vi "(SubVI)Haptic Vibration Scope.vi"() -> ()   [LabVIEW 2020]
uses:
  Controls/(Ctrl)Scope_Peak to Peak.ctl
  Controls/(Ctrl)Scope_Sensor Axis.ctl
  Controls/(Ctrl)Scope_Queue Cluster.ctl
  Controls/(Ctrl)Scope_Command Enum.ctl
  Control Data/Controls/(Ctrl)Control Data_Save or Load Control Data_Function.ctl
  Mode Event/Controls/(Ctrl)Mode Event_FGV Function.ctl
  <vilib>/Utility/miscctls.llb/LVPointTypeDef.ctl
  Mode Event/Controls/(Ctrl)Mode Event_Event Type.ctl
  Serial/Controls/(Ctrl)Serial_FGV Function.ctl
  Controls/(Ctrl)Scope_Mode.ctl
  04adf9c7-eebe-4733-9548-b5fb3f9c431f.vi
  aeb30a4b-5dd8-45a1-ad12-ebdf0f741a30.vi
  Variables/(Var)System Variables.vi
panel:
  in  "Graph_Legend Blind S3":string
  in  "Graph_Legend Blind S2":string
  in  "Graph_Legend Blind S1":string
  in  "Scope_Stop":bool
  in  "Mode":enum32{"Auto Playback", "Scope Mode"}(tab)=enum."Scope Mode"
  in  "Auto_Record Time":dbl(ring)=0.1 caption="Record Time" items=["0.1sec"=0.1, "0.2sec"=0.2, "0.3sec"=0.3, "0.4sec"=0.4, "0.5sec"=0.5]
  in  "Auto_Start":bool
  in  "Scope_Start":bool
  in  "Scope_Trig Type":enum16{"None", "Repeat", "Single"}(ring) caption="Trigger"
  in  "Scope_Trig Ch":i32(ring)=-1 caption="Channel" items=["All Channel"=-1, "Sensor 1 - X"=0, "Sensor 1 - Y"=1, "Sensor 1 - Z"=2, "Sensor 2 - X"=3, "Sensor 2 - Y"=4, "Sensor 2 - Z"=5, "Sensor 3 - X"=6, "Sensor 3 - Y"=7, "Sensor 3 - Z"=8]
  in  "Scope_Trig Level":dbl=1.0 caption="Level" min=-16.0 max=16.0 format="%#_gg"
  in  "Scope_Trig Edge":enum16{"Rising", "Falling"}(ring) caption="Edge"
  in  "Scope_Pre-trigger":dbl(ring)=0.1 caption="Pre-trigger" items=["0%"=0.0, "10%"=0.1, "20%"=0.2, "30%"=0.3, "40%"=0.4, "50%"=0.5, "60%"=0.6, "70%"=0.7, "80%"=0.8, "90%"=0.9, "100%"=1.0]
  in  "Scope_Record Time":dbl(ring)=1.0 caption="Record Time" items=["0.1sec"=0.1, "0.2sec"=0.2, "0.3sec"=0.3, "0.4sec"=0.4, "0.5sec"=0.5, "0.6sec"=0.6, "0.7sec"=0.7, "0.8sec"=0.8, "0.9sec"=0.9, "1sec"=1.0, "2sec"=2.0, "3sec"=3.0, "4sec"=4.0, "5sec"=5.0, "6sec"=6.0, "7sec"=7.0, "8sec"=8.0, "9sec"=9.0, "10sec"=10.0]
  out "Graph":dbl[][](graph)
  out "Overrun Cnt":i32
  out "Latency":i32
  out "Graph_PP":T1 {"S3_Value" format="%#_gg"; "S2_Value" format="%#_gg"; "S1_Value" format="%#_gg"}
  in  "Graph_Auto Scale_Y":enum32{"선택 없음", "±16 g", "Auto Scale"}(radio)=enum."±16 g" caption="Y (Acc) -"
  in  "Graph_Auto Scale_X":bool=TRUE
  # "Haptic Vibration Scope"
  # "Sensor 1"
  # "Sensor 2"
  # "Sensor 3"
  # "Graph Scale"
  # "P·P"
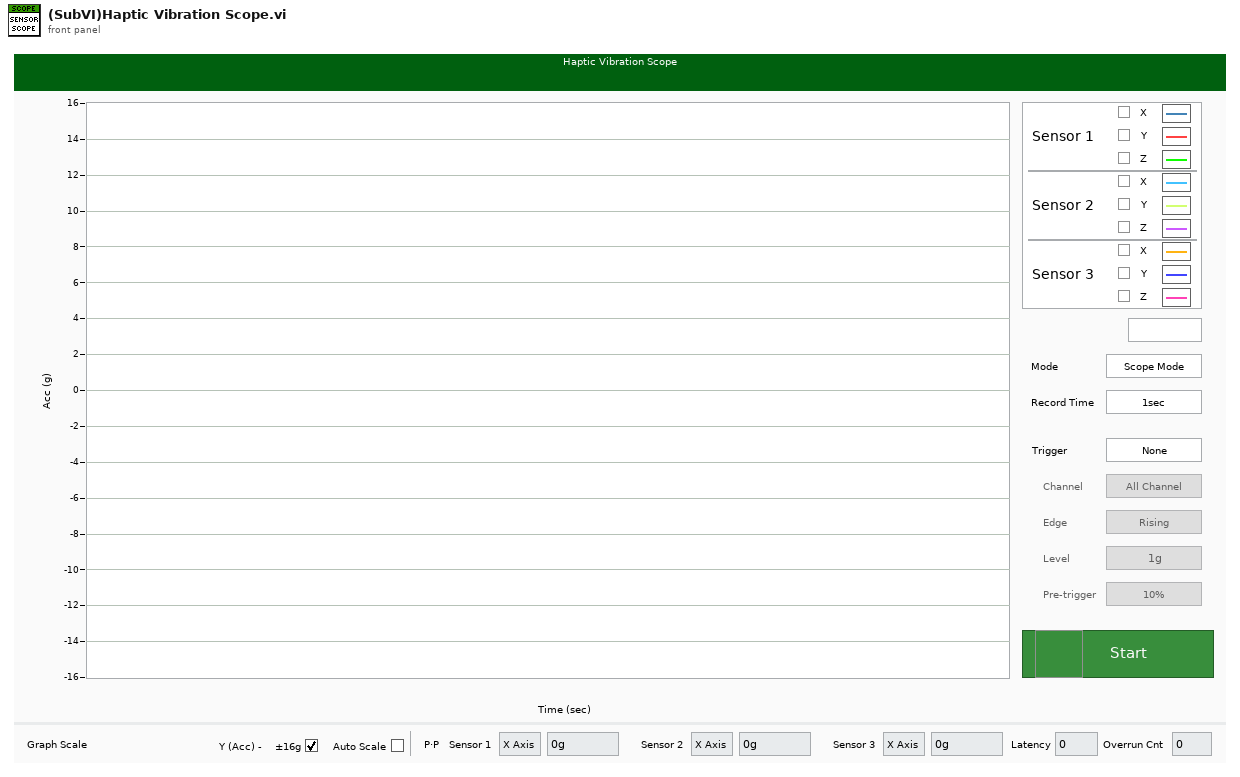
[diagram p1: front panel]
types:
  T1 = typedef "(Ctrl)Scope_Peak to Peak.ctl" = cluster{"S1_Axis":T2, "S1_Value":dbl, "S2_Axis":T2, "S2_Value":dbl, "S3_Axis":T2, "S3_Value":dbl}
  T2 = typedef "(Ctrl)Scope_Sensor Axis.ctl" = enum16{"X Axis", "Y Axis", "Z Axis"}
  T3 = enum8{"Enabled", "Disabled", "Disabled and Grayed Out"}
  T4 = typedef "(Ctrl)Mode Event_FGV Function.ctl" = enum16{"Init", "Get Event Ref", "Gen Event", "Destroy"}
  T5 = typedef "(Ctrl)Control Data_Save or Load Control Data_Function.ctl" = enum16{"Save", "Load"}
  T6 = typedef "(Ctrl)Scope_Queue Cluster.ctl" = cluster{"Command":T7, "Data":variant}
  T7 = typedef "(Ctrl)Scope_Command Enum.ctl" = enum16{"Scope_Start", "Scope_Receive", "Scope_I2C", "Scope_Stop"}
  T8 = typedef "LVPointTypeDef.ctl" = cluster{"Horizontal":i16, "Vertical":i16}
  T9 = typedef "Haptic IC.lvclass/(Ctrl)IC Type.ctl" = enum8{"DW7800", "DW7802", "DW7912", "DW7914"}
  T10 = enum32{"Page Enabled", "Page Disabled", "Page Disabled & Grayed"}
  T11 = typedef "(Ctrl)Mode Event_Event Type.ctl" = enum16{"RTP Play", "RTP Stop", "Scope Start", "Scope Stop"}
  T12 = typedef "(Ctrl)Scope_Mode.ctl" = enum8{"Auto Trigger Mode", "Continuous Mode"}
  T13 = typedef "(Ctrl)Serial_FGV Function.ctl" = enum16{"Initialize", "Read", "Read All", "Write", "Flush Buffer", "Get Ref.", "Close"}
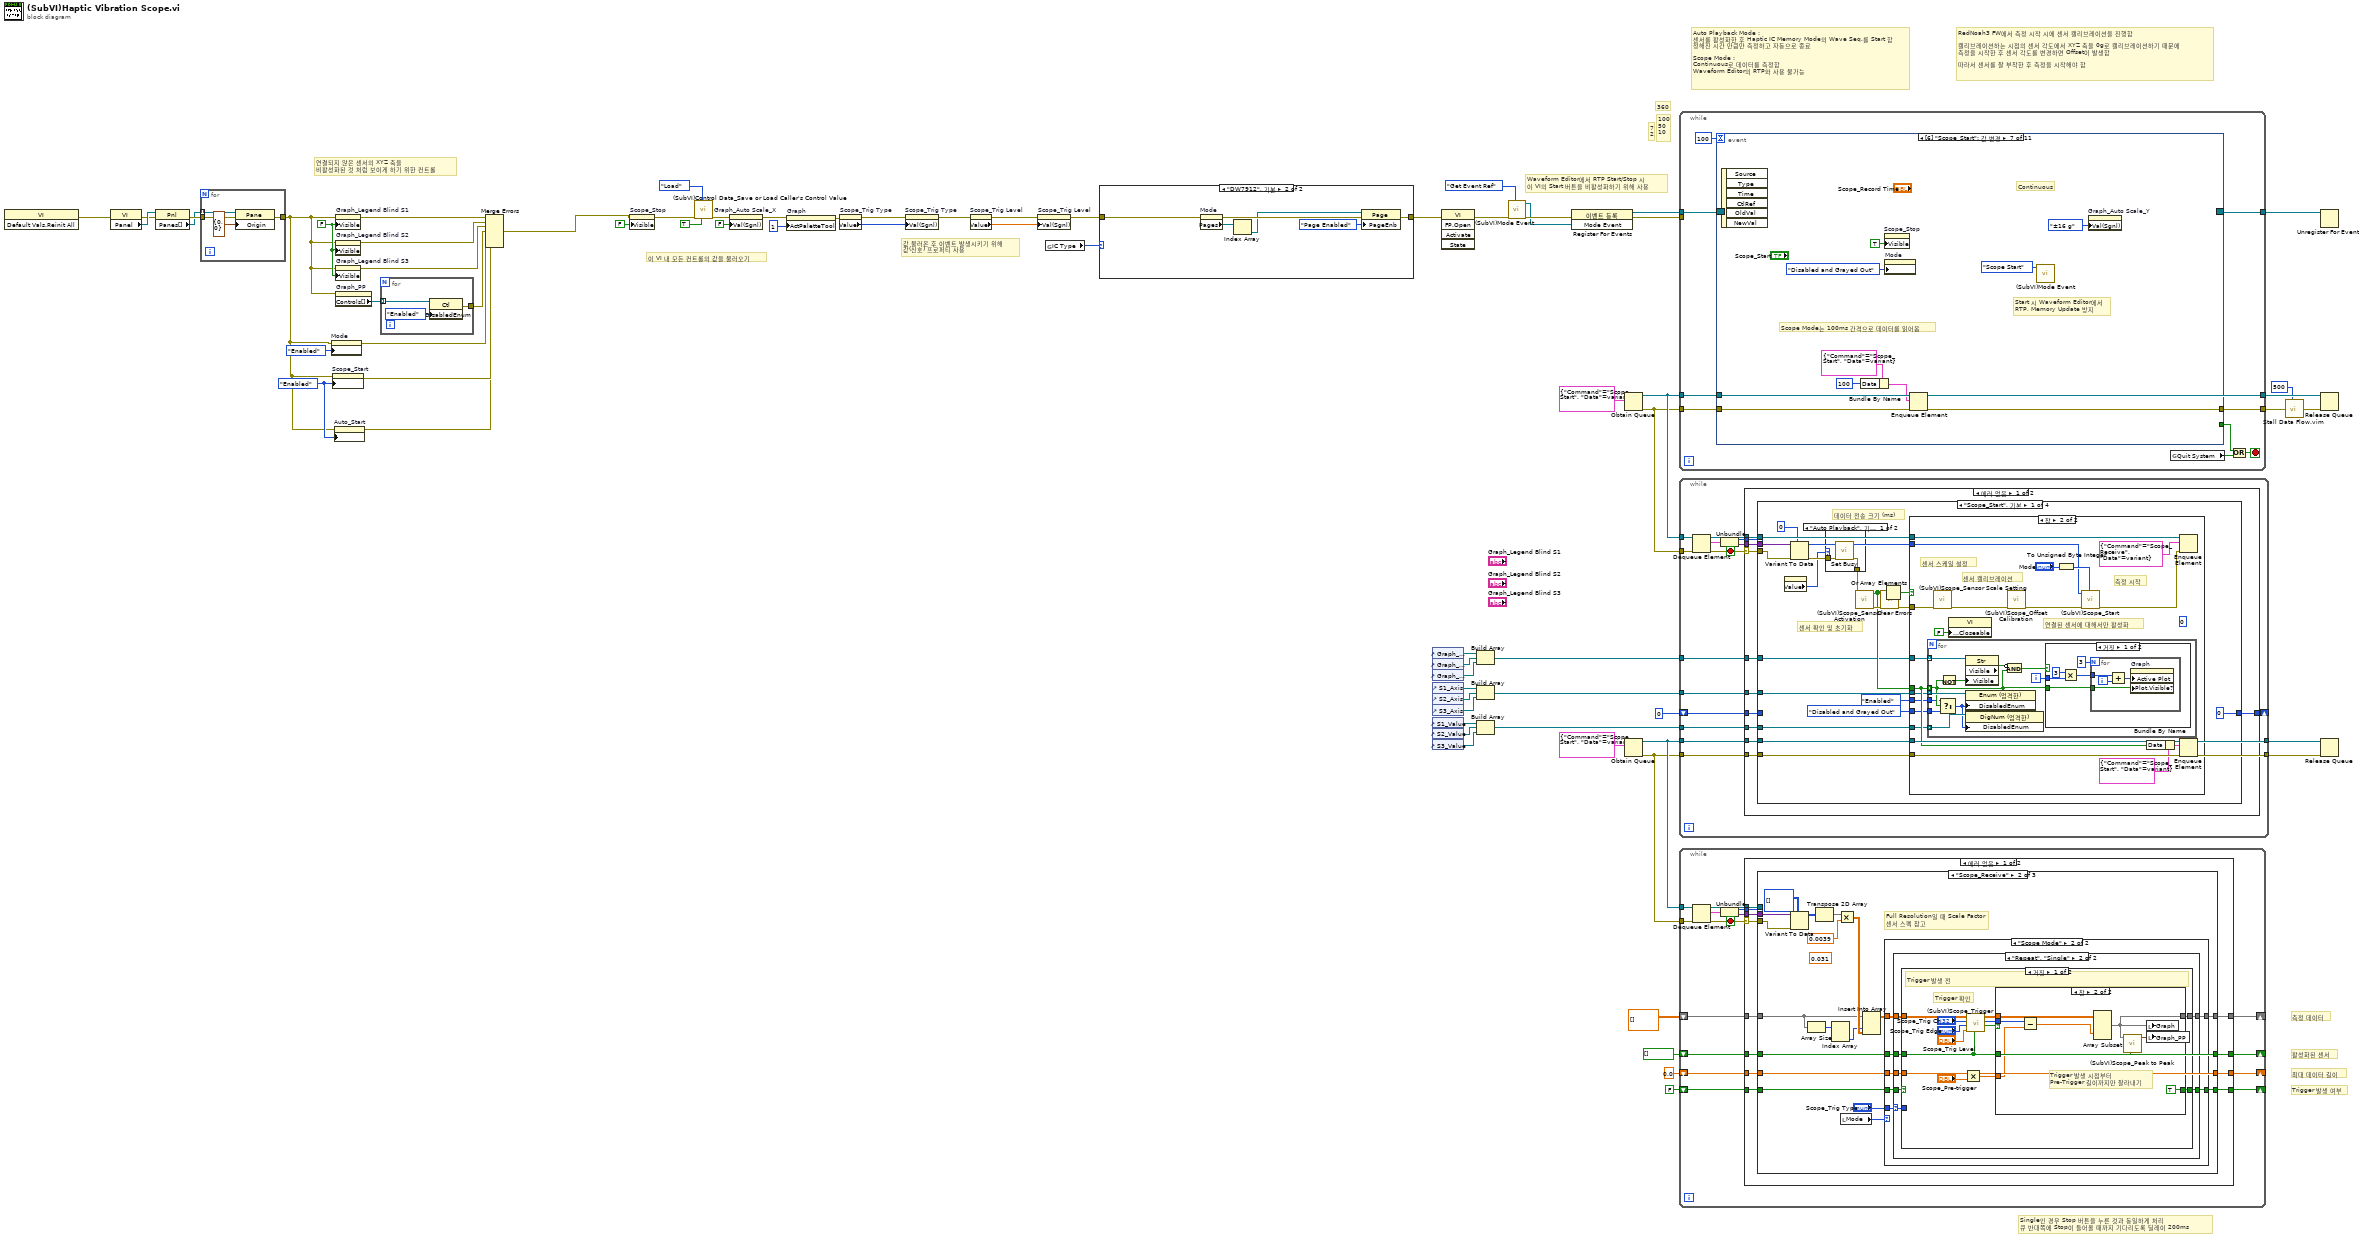
[diagram p0: block diagram]
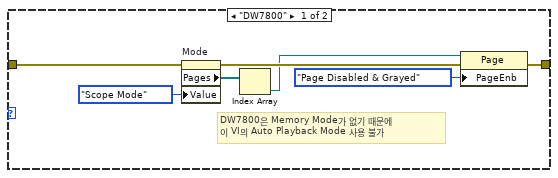
[diagram p2: hidden frame]
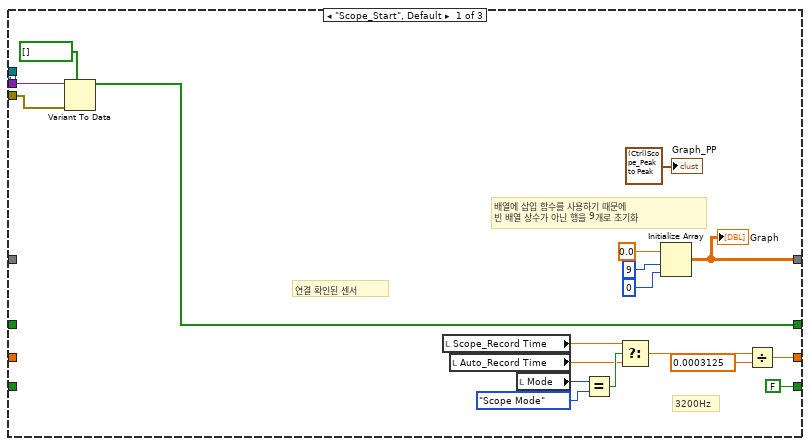
[diagram p3: hidden frame]
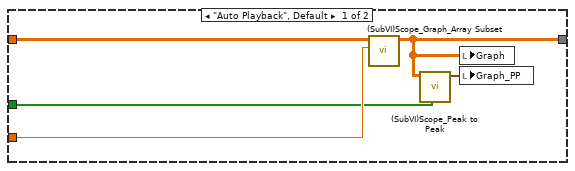
[diagram p4: hidden frame]
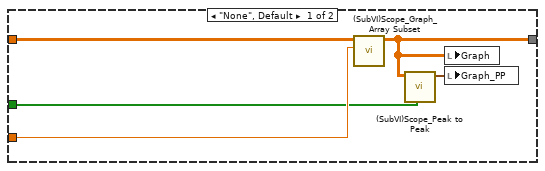
[diagram p5: hidden frame]
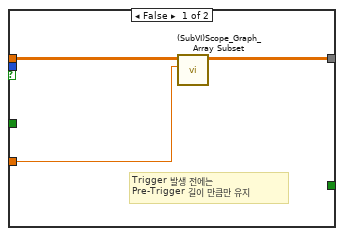
[diagram p6: hidden frame]
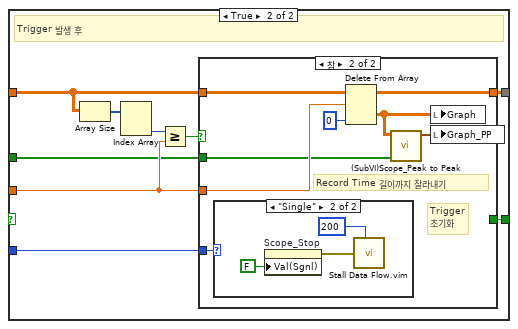
[diagram p7: hidden frame]
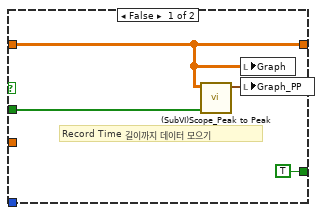
[diagram p8: hidden frame]
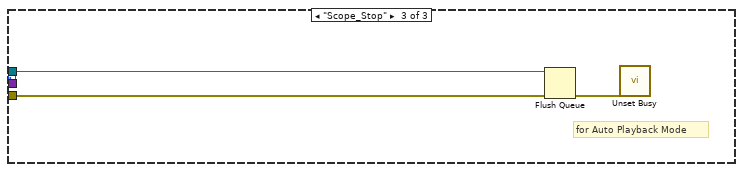
[diagram p10: hidden frame]
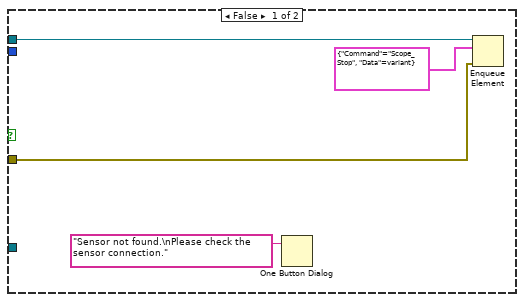
[diagram p13: hidden frame]
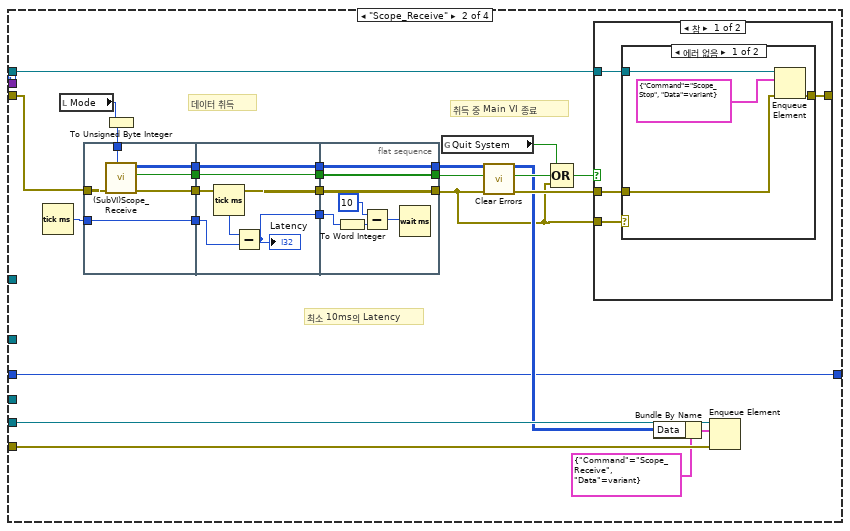
[diagram p15: hidden frame]
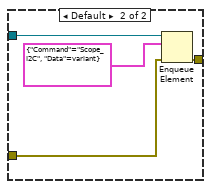
[diagram p16: hidden frame]
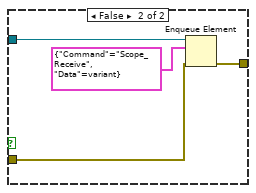
[diagram p17: hidden frame]
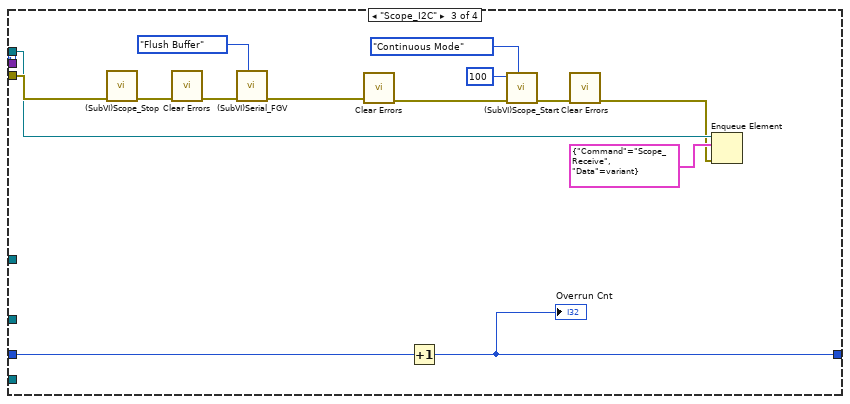
[diagram p18: hidden frame]
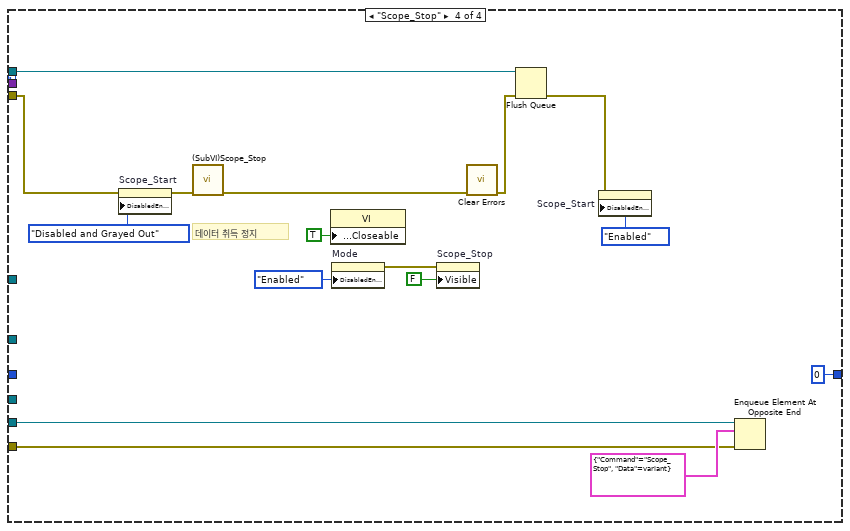
[diagram p19: hidden frame]
diagram:
  w10 = T3."Enabled" ("비활성화")
  w31 = FALSE ("보이기")
  # "7\n2"
  # "360"
  # "100\n50\n10"
  # "Single인 경우 Stop 버튼을 누른 것과 동일하게 처리\n큐 반대쪽에 Stop이 들어올 때까지 기다리도록 딜레이 200ms"
  # "Trigger 발생 여부"
  # "최대 데이터 길이"
  # "활성화된 센서"
  # "측정 데이터"
  # "RedNoah3 FW에서 측정 시작 시에 센서 캘리브레이션을 진행함\n\n캘리브레이션하는 시점의 센서 각도에서 XYZ 축을 0g로 캘리브레이션하기 때문에\n측정을 시작한 후 센서 각도를 변경하면 Offset이 발생함\n\n따라서 센서를 잘 부착한 후 측정을 시작해야 함"
  # "Auto Playback Mode : \n센서를 활성화한 후 Haptic IC Memory Mode의 Wave Seq.를 Start 함\n정해진 시간 만큼만 측정하고 자동으로 종료\n\nScope Mode : \nContinuous로 데이터를 측정함\nWaveform Editor의 RTP와 사용 불가능"
  # "Waveform Editor에서 RTP Start/Stop 시\n이 VI의 Start 버튼을 비활성화하기 위해 사용"
  # "값 불러온 후 이벤트 발생시키기 위해\n값(신호) 프로퍼티 사용"
  # "이 VI 내 모든 컨트롤의 값을 불러오기"
  # "연결되지 않은 센서의 XYZ 축을 \n비활성화된 것 처럼 보이게 하기 위한 컨트롤"
  n1 = invoke class="VI" method="Default Vals.Reinit All"() -> (error out=w35:errorcluster)  [unwired: 3 in, 2 out]
  n2 = property class="VI"(error in=w35) -> (error out=w34:errorcluster, "Panel"=w36:refnum<vi>)  [unwired: 1 in, 1 out]
  n3 = property class="Pnl"(reference=w36, error in=w34) -> (error out=w33:errorcluster, "Panes[]"=w32:refnum<vi>[])  [unwired: 1 out]
  n4 = for {
    tunnel: w33 -> [w75]
    tunnel: w32 -> [w74] mode=indexing
    tunnel: [w72] -> w9
    n5 = property class="Pane"(reference=w74, error in=w75, "Origin"=T8 {"Horizontal"=0, "Vertical"=0} ("원점")) -> (error out=w72:errorcluster)  [unwired: 1 out]
  }
  n6 = property on="Mode" class="TabCtl (엄격한)"(error in=w9, "DisabledEnum"=T3."Enabled" ("비활성화")) -> (error out=w8:errorcluster)  [unwired: 1 in, 1 out]
  n7 = property on="Scope_Start" class="Bool"(error in=w9, "DisabledEnum"=w10) -> (error out=w7:errorcluster)  [unwired: 1 in, 1 out]
  n8 = property on="Auto_Start" class="Bool"(error in=w9, "DisabledEnum"=w10) -> (error out=w6:errorcluster)  [unwired: 1 in, 1 out]
  n9 = property on="Graph_Legend Blind S1" class="Str"(error in=w9, "Visible"=w31) -> (error out=w30:errorcluster)  [unwired: 1 in, 1 out]
  n10 = property on="Graph_Legend Blind S2" class="Str"(error in=w9, "Visible"=w31) -> (error out=w29:errorcluster)  [unwired: 1 in, 1 out]
  n11 = property on="Graph_Legend Blind S3" class="Str"(error in=w9, "Visible"=w31) -> (error out=w28:errorcluster)  [unwired: 1 in, 1 out]
  n12 = property on="Graph_PP" class="Clust (엄격한)"(error in=w9) -> ("Controls[]"=w15:refnum<vi>[])  [unwired: 1 in, 2 out]
  n13 = for {
    tunnel: w15 -> [w78] mode=indexing
    tunnel: [w76] -> w14
    n14 = property class="Ctl"(reference=w78, "DisabledEnum"=T3."Enabled" ("비활성화")) -> (error out=w76:errorcluster)  [unwired: 1 in, 1 out]
  }
  n15 = Merge Errors(w30, w29, w28, w14, w8, w6, w7) -> (w1:errorcluster)
  n16 = property on="Scope_Stop" class="Bool (엄격한)"(error in=w1, "Visible"=FALSE ("보이기")) -> (error out=w64:errorcluster)  [unwired: 1 in, 1 out]
  n17 = call "(SubVI)Control Data_Save or Load Caller's Control Value.vi"("Common?"=TRUE, "Function"=(Ctrl)Control_Data_Save_or_Load_Control_Data_Function."Load", "error in (no error)"=w64) -> ("error out"=w13:errorcluster)  [unwired: 8 in]
  n18 = property on="Graph_Auto Scale_X" class="Bool (엄격한)"(error in=w13, "Val(Sgnl)"=FALSE ("값(신호)")) -> (error out=w5:errorcluster)  [unwired: 1 in, 1 out]
  n19 = property on="Graph" class="WFGraph (엄격한)"(error in=w5, "ActPaletteTool"=1 ("팔레트:활성 도구")) -> (error out=w4:errorcluster)  [unwired: 1 in, 1 out]
  n20 = property on="Scope_Trig Type" class="Enum (엄격한)"(error in=w4) -> (error out=w50:errorcluster, "Value"=w49:enum16{"None", "Repeat", "Single"})  [unwired: 1 in, 1 out]
  n21 = property on="Scope_Trig Type" class="Enum (엄격한)"(error in=w50, "Val(Sgnl)"=w49) -> (error out=w48:errorcluster)  [unwired: 1 in, 1 out]
  n22 = property on="Scope_Trig Level" class="DigNum (엄격한)"(error in=w48) -> (error out=w46:errorcluster, "Value"=w47:dbl)  [unwired: 1 in, 1 out]
  n23 = property on="Scope_Trig Level" class="DigNum (엄격한)"(error in=w46, "Val(Sgnl)"=w47) -> (error out=w45:errorcluster)  [unwired: 1 in, 1 out]
  n24 = global read "(Var)System Variables.vi" "IC Type"() -> (w51:T9)
  n25 = case shown="\"DW7912\", 기본" w51 {
    tunnel: [w82 w88] -> w63
    tunnel: w45 -> [w81 w87]
    frame "DW7800" {
      # "DW7800은 Memory Mode가 없기 때문에\n이 VI의 Auto Playback Mode 사용 불가"
      n26 = property on="Mode" class="TabCtl (엄격한)"(error in=w81, "Value"=enum32{"Auto Playback", "Scope Mode"}."Scope Mode" ("Mode")) -> (error out=w84:errorcluster, "Pages"=w85:refnum<vi>[])  [unwired: 1 in, 1 out]
      n27 = Index Array(array=w85) -> (element=w83:refnum<vi>)  [unwired: 1 in]
      n28 = property class="Page"(reference=w83, error in=w84, "PageEnb"=T10."Page Disabled & Grayed" ("페이지 활성화 상태")) -> (error out=w82:errorcluster)  [unwired: 1 out]
    }
    frame "DW7912", Default {
      n29 = property on="Mode" class="TabCtl (엄격한)"(error in=w87) -> (error out=w90:errorcluster, "Pages"=w91:refnum<vi>[])  [unwired: 1 in, 1 out]
      n30 = Index Array(array=w91) -> (element=w89:refnum<vi>)  [unwired: 1 in]
      n31 = property class="Page"(reference=w89, error in=w90, "PageEnb"=T10."Page Enabled" ("페이지 활성화 상태")) -> (error out=w88:errorcluster)  [unwired: 1 out]
    }
  }
  n32 = control-ref of="Graph_Legend Blind S1"() -> (w27:refnum<vi>)
  n33 = control-ref of="Graph_Legend Blind S2"() -> (w26:refnum<vi>)
  n34 = control-ref of="Graph_Legend Blind S3"() -> (w25:refnum<vi>)
  n35 = control-ref of="S1_Axis"() -> (w23:refnum<vi>)
  n36 = control-ref of="S2_Axis"() -> (w22:refnum<vi>)
  n37 = control-ref of="S3_Axis"() -> (w21:refnum<vi>)
  n38 = control-ref of="S1_Value"() -> (w20:refnum<vi>)
  n39 = control-ref of="S2_Value"() -> (w19:refnum<vi>)
  n40 = control-ref of="S3_Value"() -> (w18:refnum<vi>)
  n41 = invoke class="VI" method="FP.Open"(error in=w63) -> (error out=w71:errorcluster)  [unwired: 4 in, 4 out]
  n42 = Build Array(w27, w26, w25) -> (w24:refnum<vi>[])
  n43 = Build Array(w23, w22, w21) -> (w17:refnum<vi>[])
  n44 = Build Array(w20, w19, w18) -> (w16:refnum<vi>[])
  n45 = call "(SubVI)Mode Event.vi"("Function (Gen)"=(Ctrl)Mode_Event_FGV_Function."Get Event Ref" ("Function"), "error in (no error)"=w71) -> ("error out"=w44:errorcluster, "Mode Event"=w40:refnum<user-event>)  [unwired: 8 in]
  n46 = register-events(error in=w44, w40) -> (reference out=w41:refnum<event-registration>, error out=w42:errorcluster)  [unwired: 1 in]
  n47 = Obtain Queue(element data type=T6 {"Command"=enum."Scope_Start", "Data"=variant} ("클러스터")) -> (queue out=w70:refnum<queue>, error out=w69:errorcluster)  [unwired: 4 in, 1 out]
  n48 = Obtain Queue(element data type=T6 {"Command"=enum."Scope_Start", "Data"=variant} ("클러스터")) -> (queue out=w58:refnum<queue>, error out=w57:errorcluster)  [unwired: 4 in, 1 out]
  n49 = while {
    tunnel: w42 -> [_]
    tunnel: w70 -> [w95]
    tunnel: w69 -> [w94]
    tunnel: [w95] -> w68
    tunnel: [w94] -> w67
    tunnel: w41 -> [w93]
    tunnel: [w92] -> w39
    stop <- w96 stop-if-true
    n50 = event shown="[6] \"Scope_Start\": 값 변경" {
      selector: w93 -> [_ _ _ _ _ _ _ _ _ _ _]
      dyn-events: [_ _ _ _ _ _ _ _ _ _ _] -> w92
      timeout: 100 -> [_ _ _ _ _ _ _ _ _ _ _]
      tunnel: [_ TRUE _ _ _ _ _ _ _ _ _] -> w97
      tunnel: w95 -> [_ _ _ _ _ w139 w148 w153 _ _ _]
      tunnel: w94 -> [w100 _ _ _ _ w132 w145 w152 _ _ _]
      tunnel: [w100 _ _ _ _ _ _ _ _ _ _] -> _
      event Timeout {
        n51 = event-data() -> ()  [unwired: 1 in, 3 out]
      }
      event Panel Close {
        # "이 VI의 모든 컨트롤의 값을 저장"
        n52 = event-data() -> ()  [unwired: 1 in, 4 out]
        n53 = call "(SubVI)Control Data_Save or Load Caller's Control Value.vi"("Common?"=TRUE, "Function"=(Ctrl)Control_Data_Save_or_Load_Control_Data_Function."Save") -> ()  [unwired: 9 in, 1 out]
      }
      event "Scope_Trig Type", "Mode": Value Change {
        # "그래프에 Trigger 타이밍, 기준 값을 커서로 표시"
        n54 = event-data() -> ()  [unwired: 1 in, 6 out]
        n55 = local read "Scope_Record Time"() -> (w107:dbl)
        n56 = local read "Auto_Record Time"() -> (w106:dbl)
        n57 = local read "Scope_Trig Type"() -> (w112:enum16{"None", "Repeat", "Single"})
        n58 = local read "Mode"() -> (w110:enum32{"Auto Playback", "Scope Mode"})
        n59 = Not Equal?(x=w112, y=enum16{"None", "Repeat", "Single"}."None") -> (x != y?=w113:bool)
        n60 = Equal?(x=w110, y=enum32{"Auto Playback", "Scope Mode"}."Scope Mode") -> (x = y?=w108:bool)
        n61 = And(x=w113, y=w108) -> (x .and. y?=w111:bool)
        n62 = Select(t=w107, s=w108, f=w106) -> (s? t:f=w105:dbl)
        n63 = property on="Graph" class="WFGraph (엄격한)"("Cursor.Visible"=w111, "XScale.Maximum"=w105, "XScale.Minimum"=0.0 ("X 스케일.범위:최소값")) -> ()  [unwired: 2 in, 2 out]
        n64 = Select(t=T3."Enabled", s=w111, f=T3."Disabled and Grayed Out") -> (s? t:f=w114:T3)
        n65 = property on="Scope_Trig Ch" class="Ring (엄격한)"("DisabledEnum"=w114) -> ()  [unwired: 2 in, 2 out]
        n66 = property on="Scope_Trig Edge" class="Enum (엄격한)"("DisabledEnum"=w114) -> ()  [unwired: 2 in, 2 out]
        n67 = property on="Scope_Trig Level" class="DigNum (엄격한)"("DisabledEnum"=w114) -> ()  [unwired: 2 in, 2 out]
        n68 = property on="Scope_Pre-trigger" class="Ring (엄격한)"("DisabledEnum"=w114) -> ()  [unwired: 2 in, 2 out]
      }
      event "Auto_Record Time", "Scope_Record Time": Value Change {
        n69 = event-data() -> ("NewVal"=w126:dbl)  [unwired: 1 in, 5 out]
        n70 = local read "Scope_Trig Type"() -> (w122:enum16{"None", "Repeat", "Single"})
        n71 = property on="Graph" class="WFGraph (엄격한)"("XScale.Maximum"=w126, "XScale.Minimum"=0.0 ("X 스케일.범위:최소값")) -> ()  [unwired: 2 in, 2 out]
        n72 = local read "Mode"() -> (w124:enum32{"Auto Playback", "Scope Mode"})
        n73 = Equal?(x=w124, y=enum32{"Auto Playback", "Scope Mode"}."Scope Mode") -> (x = y?=w120:bool)
        n74 = Not Equal?(x=w122, y=enum16{"None", "Repeat", "Single"}."None") -> (x != y?=w119:bool)
        n75 = And(x=w120, y=w119) -> (x .and. y?=w118:bool)
        n76 = case shown="참" w118 {
          frame False {
          }
          frame True {
            # "Trigger가 활성화된 경우\nRecord Time을 변경하면\n커서 위치도 변경되어야 해서\n이벤트 발생시킴"
            n77 = local read "Scope_Pre-trigger"() -> (w127:dbl)
            n78 = property on="Scope_Pre-trigger" class="Ring (엄격한)"("Val(Sgnl)"=w127) -> ()  [unwired: 2 in, 2 out]
          }
        }
      }
      event "Scope_Trig Level", "Scope_Pre-trigger": Value Change {
        # "그래프에 Trigger 타이밍, 기준 값을 커서로 표시"
        n79 = event-data() -> ()  [unwired: 1 in, 6 out]
        n80 = local read "Scope_Record Time"() -> (w130:dbl)
        n81 = local read "Scope_Pre-trigger"() -> (w129:dbl)
        n82 = local read "Scope_Trig Level"() -> (w131:dbl)
        n83 = Compound Arithmetic op=MULTIPLY(w130, w129) -> (w128:dbl)
        n84 = property on="Graph" class="WFGraph (엄격한)"("Cursor.Cursor Y"=w131, "Cursor.Cursor X"=w128) -> ()  [unwired: 2 in, 2 out]
      }
      event "Auto_Start": Value Change {
        # "Finite\n\n측정 시작과 동시에 IC의 Memory Mode를 Play"
        # "Auto Playback Mode는 \nRecord Time 만큼의 데이터를 한번에 읽어옴"
        n85 = event-data() -> ()  [unwired: 1 in, 6 out]
        n86 = local read "Auto_Record Time"() -> (w137:dbl)
        n87 = Multiply(x=w137, y=1000.0) -> (x*y=w135:dbl)
        n88 = Bundle By Name(cluster=T6 {"Command"=enum."Scope_Start", "Data"=variant} ("원소"), "Data"=w135) -> (w136:T6)
        n89 = Enqueue Element(queue=w139, element=w136, error in (no error)=w132) -> ()  [unwired: 1 in, 3 out]
        n90 = property on="Graph_Auto Scale_Y" class="RadioBtnsControl (엄격한)"("Val(Sgnl)"=enum32{"선택 없음", "±16 g", "Auto Scale"}."±16 g" ("값(신호)")) -> ()  [unwired: 2 in, 2 out]
      }
      event "Scope_Start": Value Change {
        # "Continuous"
        # "Start 시 Waveform Editor에서 \nRTP, Memory Update 방지"
        # "Scope Mode는 100ms 간격으로 데이터를 읽어옴"
        n91 = event-data() -> ()  [unwired: 1 in, 6 out]
        n92 = Bundle By Name(cluster=T6 {"Command"=enum."Scope_Start", "Data"=variant} ("원소"), "Data"=u16 100) -> (w146:T6)
        n93 = property on="Scope_Stop" class="Bool (엄격한)"("Visible"=TRUE ("보이기")) -> ()  [unwired: 2 in, 2 out]
        n94 = property on="Mode" class="TabCtl (엄격한)"("DisabledEnum"=T3."Disabled and Grayed Out" ("비활성화")) -> ()  [unwired: 2 in, 2 out]
        n95 = Enqueue Element(queue=w148, element=w146, error in (no error)=w145) -> ()  [unwired: 1 in, 3 out]
        n96 = call "(SubVI)Mode Event.vi"("Event Type"=(Ctrl)Mode_Event_Event_Type."Scope Start") -> ()  [unwired: 9 in, 2 out]
        n97 = property on="Graph_Auto Scale_Y" class="RadioBtnsControl (엄격한)"("Val(Sgnl)"=enum32{"선택 없음", "±16 g", "Auto Scale"}."±16 g" ("값(신호)")) -> ()  [unwired: 2 in, 2 out]
      }
      event "Scope_Stop": Value Change {
        # "반대쪽에 추가해서 우선 실행되게 함"
        # "Scope Mode 종료"
        # "값(신호) 프로퍼티 사용하기 위해\n스위치 모드로 사용"
        # "Stop 시 Waveform Editor에서 \nRTP, Memory Update 가능하도록 설정"
        n98 = event-data() -> ()  [unwired: 1 in, 6 out]
        n99 = local write "Scope_Stop"(FALSE ("Scope_Stop")) -> ()
        n100 = Enqueue Element At Opposite End(queue=w153, element=T6 {"Command"=enum."Scope_Stop", "Data"=variant} ("원소"), error in (no error)=w152) -> ()  [unwired: 1 in, 3 out]
        n101 = call "(SubVI)Mode Event.vi"("Event Type"=(Ctrl)Mode_Event_Event_Type."Scope Stop") -> ()  [unwired: 9 in, 2 out]
      }
      event User Event {
        # "Waveform Editor에서 RTP Start 시 Start 버튼 비활성화\nWaveform Editor에서 RTP Stop 시 Start 버튼 활성화"
        n102 = event-data() -> ("Mode Event"=w154:T11)  [unwired: 1 in, 4 out]
        n103 = case shown="\"RTP Play\"" w154 {
          frame "RTP Play" {
            w155 = T3."Disabled and Grayed Out" ("비활성화")
            n104 = property on="Scope_Start" class="Bool"("DisabledEnum"=w155) -> ()  [unwired: 2 in, 2 out]
            n105 = property on="Auto_Start" class="Bool"("DisabledEnum"=w155) -> ()  [unwired: 2 in, 2 out]
          }
          frame "RTP Stop" {
            w156 = T3."Enabled" ("비활성화")
            n106 = property on="Scope_Start" class="Bool"("DisabledEnum"=w156) -> ()  [unwired: 2 in, 2 out]
            n107 = property on="Auto_Start" class="Bool"("DisabledEnum"=w156) -> ()  [unwired: 2 in, 2 out]
          }
          frame "Scope Start", Default {
          }
        }
      }
      event "Graph_Auto Scale_X", "Graph_Auto Scale_Y": Value Change {
        # "LabVIEW의 오토스케일이 아니라\n설정한 Record Time 범위로 설정"
        n108 = event-data() -> ("CtlRef"=w166:refnum<vi>, "OldVal"=w164:variant)  [unwired: 1 in]
        n109 = control-ref of="Graph_Auto Scale_Y"() -> (w167:refnum<vi>)
        n110 = Equal?(x=w166, y=w167) -> (x = y?=w165:bool)
        n111 = case shown="\"선택 없음\"" "Graph_Auto Scale_Y" {
          tunnel: w165 -> [w170 _ _]
          tunnel: w164 -> [w169 _ _]
          frame "선택 없음" {
            n112 = case shown="참" w170 {
              tunnel: w169 -> [_ w173]
              frame False {
              }
              frame True {
                n113 = Variant To Data(type=enum32{"선택 없음", "±16 g", "Auto Scale"}."±16 g" ("Graph_Auto Scale_Y"), Variant=w173) -> (data=w171:enum32{"선택 없음", "±16 g", "Auto Scale"})  [unwired: 1 in, 1 out]
                n114 = case shown="\"선택 없음\", 기본" w171 {
                  frame "선택 없음", Default {
                    n115 = property on="Graph" class="WFGraph (엄격한)"("YScale.ScaleFit"=u8 0 ("Y 스케일.스케일 맞춤"), "YScale.Maximum"=16.0 ("Y 스케일.범위:최대값"), "YScale.Minimum"=-16.0 ("Y 스케일.범위:최소값")) -> ()  [unwired: 2 in, 2 out]
                    n116 = property on="Graph_Auto Scale_Y" class="RadioBtnsControl (엄격한)"("Value"=enum32{"선택 없음", "±16 g", "Auto Scale"}."±16 g" ("Graph_Auto Scale_Y")) -> ()  [unwired: 2 in, 2 out]
                  }
                  frame "±16 g" {
                    n117 = property on="Graph" class="WFGraph (엄격한)"("YScale.ScaleFit"=u8 2 ("Y 스케일.스케일 맞춤")) -> ()  [unwired: 2 in, 2 out]
                    n118 = property on="Graph_Auto Scale_Y" class="RadioBtnsControl (엄격한)"("Value"=enum32{"선택 없음", "±16 g", "Auto Scale"}."Auto Scale" ("Graph_Auto Scale_Y")) -> ()  [unwired: 2 in, 2 out]
                  }
                }
              }
            }
          }
          frame "±16 g" {
            n119 = property on="Graph" class="WFGraph (엄격한)"("YScale.ScaleFit"=u8 0 ("Y 스케일.스케일 맞춤"), "YScale.Maximum"=16.0 ("Y 스케일.범위:최대값"), "YScale.Minimum"=-16.0 ("Y 스케일.범위:최소값")) -> ()  [unwired: 2 in, 2 out]
          }
          frame "Auto Scale" {
            # "LabVIEW의 오토스케일 사용"
            n120 = property on="Graph" class="WFGraph (엄격한)"("YScale.ScaleFit"=u8 2 ("Y 스케일.스케일 맞춤")) -> ()  [unwired: 2 in, 2 out]
          }
        }
        n121 = local read "Scope_Record Time"() -> (w160:dbl)
        n122 = local read "Auto_Record Time"() -> (w159:dbl)
        n123 = local read "Mode"() -> (w161:enum32{"Auto Playback", "Scope Mode"})
        n124 = Equal?(x=w161, y=enum32{"Auto Playback", "Scope Mode"}."Scope Mode") -> (x = y?=w162:bool)
        n125 = Select(t=w160, s=w162, f=w159) -> (s? t:f=w157:dbl)
        n126 = property on="Graph" class="WFGraph (엄격한)"("XScale.Maximum"=w157, "XScale.Minimum"=0.0 ("X 스케일.범위:최소값")) -> ()  [unwired: 2 in, 2 out]
      }
      event "Graph": Scale Range Change {
        # "사용자가 그래프의 스케일을 변경하는 경우\n오토스케일 관련 컨트롤 값 변경"
        n127 = event-data() -> ("Kind"=w185:enum16{"X-Scale", "Y-Scale", "Z-Scale"}, "ScaleRef"=w187:refnum<vi>)  [unwired: 1 in, 6 out]
        n128 = property class="GrphScl"(reference=w187, "ScaleFit"=u8 0 ("스케일 맞춤")) -> (error out=w184:errorcluster)  [unwired: 1 in, 1 out]
        n129 = case shown="\"Y-Scale\"" w185 {
          tunnel: w184 -> [_ _]
          frame "X-Scale", Default {
            n130 = local write "Graph_Auto Scale_X"(FALSE ("Graph_Auto Scale_X")) -> ()
          }
          frame "Y-Scale" {
            n131 = local write "Graph_Auto Scale_Y"(enum32{"선택 없음", "±16 g", "Auto Scale"}."선택 없음" ("Graph_Auto Scale_Y")) -> ()
          }
        }
      }
    }
    n132 = global read "(Var)System Variables.vi" "Quit System"() -> (w98:bool)
    n133 = Or(x=w97, y=w98) -> (x .or. y?=w96:bool)
  }
  n134 = while {
    tunnel: w70 -> [w203]
    tunnel: w69 -> [w202]
    tunnel: w58 -> [w196]
    tunnel: w57 -> [w195]
    tunnel: [w196] -> w60
    tunnel: [w195] -> w59
    tunnel: w24 -> [w194]
    tunnel: w17 -> [w193]
    tunnel: w16 -> [w192]
    shift-right: [w191] -> _
    shift-left: 0 -> [w190]
    stop <- w201 stop-if-true
    n135 = Dequeue Element(queue=w203, error in (no error)=w202) -> (queue out=w200:refnum<queue>, element=w199:T6, error out=w201:errorcluster)  [unwired: 1 in, 1 out]
    n136 = Unbundle(w199) -> ("Command"=w198:T7, "Data"=w197:variant)
    n137 = case shown="에러 없음" w201 {
      selector: w201 -> [w214 _]
      tunnel: w200 -> [w213 _]
      tunnel: w198 -> [w212 _]
      tunnel: w197 -> [w211 _]
      tunnel: w196 -> [w210 _]
      tunnel: w195 -> [w209 _]
      tunnel: w194 -> [w208 _]
      tunnel: w193 -> [w207 _]
      tunnel: w192 -> [w206 _]
      tunnel: [w205 w371] -> w191
      tunnel: w190 -> [w204 w371]
      frame No Error {
        n138 = case shown="\"Scope_Start\", 기본" w212 {
          tunnel: w214 -> [w231 w288 w353 w360]
          tunnel: w213 -> [w233 w305 w352 w370]
          tunnel: w211 -> [w232 _ _ _]
          tunnel: w210 -> [w228 w301 _ w365]
          tunnel: w209 -> [w227 w300 _ w364]
          tunnel: w208 -> [w224 _ _ _]
          tunnel: w207 -> [w223 _ _ _]
          tunnel: w206 -> [w222 _ _ _]
          tunnel: [0 w282 w350 0] -> w205
          tunnel: w204 -> [_ w282 w351 _]
          frame "Scope_Start", Default {
            # "데이터 전송 크기 (ms)"
            # "센서 확인 및 초기화"
            n139 = property class="Enum (엄격한)"() -> ("Value"=w215:enum32{"Auto Playback", "Scope Mode"})  [unwired: 2 in, 2 out]
            n140 = Variant To Data(error in=w231, type=u16 0 ("타입"), Variant=w232) -> (data=w229:u16, error out=w216:errorcluster)
            n141 = case shown="\"Auto Playback\", 기본" w215 {
              tunnel: [w236 w237] -> w217
              tunnel: w216 -> [w235 w237]
              frame "Auto Playback", Default {
                n142 = call <vilib>:"Set Busy.vi"("error in (no error)"=w235) -> ("error out"=w236:errorcluster)  [unwired: 9 in, 1 out]
              }
              frame "Scope Mode" {
              }
            }
            n143 = call "(SubVI)Scope_Sensor Activation.vi"("error in (no error)"=w217) -> ("error out"=w234:errorcluster, "Valid"=w226:bool[])  [unwired: 9 in]
            n144 = call <vilib>:"Clear Errors.vi"("error in (no error)"=w234) -> ("error out"=w219:errorcluster)  [unwired: 5 in, 1 out]
            n145 = Or Array Elements(Boolean array=w226) -> (logical OR=w225:bool)
            n146 = case shown="참" w225 {
              tunnel: w219 -> [w239 w259]
              tunnel: w233 -> [w240 w257]
              tunnel: w229 -> [_ w254]
              tunnel: w228 -> [_ w251]
              tunnel: w227 -> [_ w250]
              tunnel: w226 -> [_ w247]
              tunnel: w224 -> [_ w246]
              tunnel: w223 -> [_ w245]
              tunnel: w222 -> [_ w244]
              tunnel: T3."Enabled" ("비활성화") -> [_ w243]
              tunnel: T3."Disabled and Grayed Out" ("비활성화") -> [_ w242]
              frame False {
                n147 = One Button Dialog(message="Sensor not found.\nPlease check the sensor connection." ("메시지")) -> ()  [unwired: 1 in, 1 out]
                n148 = Enqueue Element(queue=w240, element=T6 {"Command"=enum."Scope_Stop", "Data"=variant} ("클러스터"), error in (no error)=w239) -> ()  [unwired: 1 in, 3 out]
              }
              frame True {
                (unwired) 0
                # "측정 시작"
                # "센서 캘리브레이션"
                # "센서 스케일 설정"
                # "연결된 센서에 대해서만 활성화"
                n149 = for {
                  tunnel: w247 -> [w265] mode=indexing
                  tunnel: w246 -> [w271] mode=indexing
                  tunnel: w245 -> [w267] mode=indexing
                  tunnel: w244 -> [w266] mode=indexing
                  tunnel: w243 -> [w264]
                  tunnel: w242 -> [w263]
                  i -> [w272]
                  n150 = Select(t=w264, s=w265, f=w263) -> (s? t:f=w262:T3)
                  n151 = Not(x=w265) -> (.not. x?=w270:bool)
                  n152 = property class="Str"(reference=w271, "Visible"=w270) -> ("Visible"=w269:bool)  [unwired: 1 in, 2 out]
                  n153 = property class="Enum (엄격한)"(reference=w267, "DisabledEnum"=w262) -> ()  [unwired: 1 in, 2 out]
                  n154 = property class="DigNum (엄격한)"(reference=w266, "DisabledEnum"=w262) -> ()  [unwired: 1 in, 2 out]
                  n155 = Compound Arithmetic op=AND(invert w269, w265) -> (w268:bool)
                  n156 = case shown="거짓" w268 {
                    tunnel: w272 -> [w277 _]
                    tunnel: w265 -> [w273 _]
                    frame False {
                      n157 = Multiply(x=3 ("y"), y=w277) -> (x*y=w275:i32)
                      n158 = for {
                        N: 3 -> [_]
                        tunnel: w275 -> [w281]
                        tunnel: w273 -> [w278]
                        i -> [w280]
                        n159 = Add(x=w281, y=w280) -> (x+y=w279:i32)
                        n160 = property on="Graph" class="WFGraph (엄격한)"("Active Plot"=w279, "Plot.Visible?"=w278) -> ()  [unwired: 2 in, 2 out]
                      }
                    }
                    frame True {
                    }
                  }
                }
                n161 = call "(SubVI)Scope_Sensor Scale Setting.vi"("error in (no error)"=w259) -> ("error out"=w260:errorcluster)  [unwired: 9 in]
                n162 = property class="VI"("Front Panel.Closeable"=FALSE ("프런트패널 윈도우:닫기 가능")) -> ()  [unwired: 2 in, 2 out]
                n163 = call "(SubVI)Scope_Offset Calibration.vi"("error in (no error)"=w260) -> ("error out"=w261:errorcluster)  [unwired: 10 in]
                n164 = To Unsigned Byte Integer(number="Mode") -> (unsigned 8bit integer=w256:u8)
                n165 = call "(SubVI)Scope_Start.vi"("Mode"=w256, "error in (no error)"=w261, "Recording Time"=w254) -> ("error out"=w258:errorcluster)  [unwired: 8 in]
                n166 = Bundle By Name(cluster=T6 {"Command"=enum."Scope_Start", "Data"=variant} ("클러스터"), "Data"=w247) -> (w248:T6)
                n167 = Enqueue Element(queue=w257, element=T6 {"Command"=enum."Scope_Receive", "Data"=variant} ("클러스터"), error in (no error)=w258) -> ()  [unwired: 1 in, 3 out]
                n168 = Enqueue Element(queue=w251, element=w248, error in (no error)=w250) -> ()  [unwired: 1 in, 3 out]
              }
            }
          }
          frame "Scope_Receive" {
            # "최소 10ms의 Latency"
            # "데이터 취득"
            # "취득 중 Main VI 종료"
            n169 = Tick Count (ms)() -> (millisecond timer value=w289:u32)
            n170 = local read "Mode"() -> (w304:enum32{"Auto Playback", "Scope Mode"})
            n171 = flat-sequence {
              tunnel: w288 -> [w311]
              tunnel: w303 -> [w309]
              tunnel: [w310] -> w293
              tunnel: [w308] -> w292
              tunnel: [w307] -> w291
              tunnel: w289 -> [w306]
              tunnel: [w306] -> w290
              tunnel: w293 -> [w317]
              tunnel: w292 -> [w316]
              tunnel: w291 -> [w315]
              tunnel: w290 -> [w313]
              tunnel: [w317] -> w287
              tunnel: [w316] -> w286
              tunnel: [w315] -> w285
              tunnel: [w312] -> w284
              tunnel: [w322] -> w294
              tunnel: [w323] -> w302
              tunnel: [w324] -> w283
              tunnel: w287 -> [w324]
              tunnel: w286 -> [w323]
              tunnel: w285 -> [w322]
              tunnel: w284 -> [w319]
              frame #0 {
                n172 = call "(SubVI)Scope_Receive.vi"("User Code"=w309, "error in (no error)"=w311) -> ("error out"=w310:errorcluster, "End"=w308:bool, "Data"=w307:i16[][])  [unwired: 7 in]
              }
              frame #1 {
                n173 = Tick Count (ms)() -> (millisecond timer value=w314:u32)
                n174 = Subtract(x=w314, y=w313) -> (x-y=w312:u32)
                "Latency" <- w312
              }
              frame #2 {
                n175 = To Word Integer(number=w319) -> (16bit integer=w318:i16)
                n176 = Subtract(x=10 ("x-y"), y=w318) -> (x-y=w321:i32)
                n177 = Wait (ms)(milliseconds to wait=w321) -> ()  [unwired: 1 out]
              }
            }
            n178 = To Unsigned Byte Integer(number=w304) -> (unsigned 8bit integer=w303:u8)
            n179 = global read "(Var)System Variables.vi" "Quit System"() -> (w296:bool)
            n180 = call <vilib>:"Clear Errors.vi"("error in (no error)"=w283) -> ("error out"=w295:errorcluster)  [unwired: 5 in, 1 out]
            n181 = Compound Arithmetic op=OR(w296, w302, w283) -> (w297:bool)
            n182 = case shown="참" w297 {
              tunnel: w305 -> [w328 w340]
              tunnel: w295 -> [w327 w337]
              tunnel: [w326 w338] -> _
              tunnel: w283 -> [w325 _]
              frame True {
                n183 = case shown="에러 없음" w325 {
                  tunnel: w328 -> [w332 w336]
                  tunnel: w327 -> [w330 w334]
                  tunnel: [w329 w333] -> w326
                  frame No Error {
                    n184 = Enqueue Element(queue=w332, element=T6 {"Command"=enum."Scope_Stop", "Data"=variant} ("클러스터"), error in (no error)=w330) -> (error out=w329:errorcluster)  [unwired: 1 in, 2 out]
                  }
                  frame Default {
                    n185 = Enqueue Element(queue=w336, element=T6 {"Command"=enum."Scope_I2C", "Data"=variant} ("클러스터"), error in (no error)=w334) -> (error out=w333:errorcluster)  [unwired: 1 in, 2 out]
                  }
                }
              }
              frame False {
                n186 = Enqueue Element(queue=w340, element=T6 {"Command"=enum."Scope_Receive", "Data"=variant} ("클러스터"), error in (no error)=w337) -> (error out=w338:errorcluster)  [unwired: 1 in, 2 out]
              }
            }
            n187 = Bundle By Name(cluster=T6 {"Command"=enum."Scope_Receive", "Data"=variant} ("클러스터"), "Data"=w294) -> (w298:T6)
            n188 = Enqueue Element(queue=w301, element=w298, error in (no error)=w300) -> ()  [unwired: 1 in, 3 out]
          }
          frame "Scope_I2C" {
            n189 = call "(SubVI)Scope_Stop.vi"("error in (no error)"=w353) -> ("error out"=w348:errorcluster)  [unwired: 10 in]
            n190 = call <vilib>:"Clear Errors.vi"("error in (no error)"=w348) -> ("error out"=w341:errorcluster)  [unwired: 5 in, 1 out]
            n191 = call "(SubVI)Serial_FGV.vi"("Function"=(Ctrl)Serial_FGV_Function."Flush Buffer", "error in (no error)"=w341) -> ("error out"=w347:errorcluster)  [unwired: 7 in, 2 out]
            n192 = call <vilib>:"Clear Errors.vi"("error in (no error)"=w347) -> ("error out"=w345:errorcluster)  [unwired: 5 in, 1 out]
            n193 = Increment(x=w351) -> (x+1=w350:i32)
            "Overrun Cnt" <- w350
            n194 = call "(SubVI)Scope_Start.vi"("Mode"=(Ctrl)Scope_Mode."Continuous Mode", "error in (no error)"=w345, "Recording Time"=u16 100) -> ("error out"=w344:errorcluster)  [unwired: 8 in]
            n195 = call <vilib>:"Clear Errors.vi"("error in (no error)"=w344) -> ("error out"=w349:errorcluster)  [unwired: 5 in, 1 out]
            n196 = Enqueue Element(queue=w352, element=T6 {"Command"=enum."Scope_Receive", "Data"=variant} ("클러스터"), error in (no error)=w349) -> ()  [unwired: 1 in, 3 out]
          }
          frame "Scope_Stop" {
            # "데이터 취득 정지"
            n197 = property on="Scope_Start" class="Bool"(error in=w360, "DisabledEnum"=T3."Disabled and Grayed Out" ("비활성화")) -> (error out=w359:errorcluster)  [unwired: 1 in, 1 out]
            n198 = call "(SubVI)Scope_Stop.vi"("error in (no error)"=w359) -> ("error out"=w362:errorcluster)  [unwired: 10 in]
            n199 = property class="VI"("Front Panel.Closeable"=TRUE ("프런트패널 윈도우:닫기 가능")) -> ()  [unwired: 2 in, 2 out]
            n200 = property on="Mode" class="TabCtl (엄격한)"("DisabledEnum"=T3."Enabled" ("비활성화")) -> (error out=w363:errorcluster)  [unwired: 2 in, 1 out]
            n201 = property on="Scope_Stop" class="Bool (엄격한)"(error in=w363, "Visible"=FALSE ("보이기")) -> ()  [unwired: 1 in, 2 out]
            n202 = call <vilib>:"Clear Errors.vi"("error in (no error)"=w362) -> ("error out"=w356:errorcluster)  [unwired: 5 in, 1 out]
            n203 = Flush Queue(queue=w370, error in (no error)=w356) -> (error out=w355:errorcluster)  [unwired: 2 out]
            n204 = property on="Scope_Start" class="Bool"(error in=w355, "DisabledEnum"=T3."Enabled" ("비활성화")) -> ()  [unwired: 1 in, 2 out]
            n205 = Enqueue Element At Opposite End(queue=w365, element=T6 {"Command"=enum."Scope_Stop", "Data"=variant} ("클러스터"), error in (no error)=w364) -> ()  [unwired: 1 in, 3 out]
          }
        }
      }
      frame Error {
      }
    }
  }
  n206 = while {
    tunnel: w58 -> [w386]
    tunnel: w57 -> [w385]
    shift-right: [w379] -> _
    shift-left: dbl[][] [] ("x*y") -> [w378]
    shift-right: [w377] -> _
    shift-left: 0.0 -> [w376]
    shift-right: [w375] -> _
    shift-left: FALSE -> [w374]
    shift-right: [w373] -> _
    shift-left: bool[] [] ("타입") -> [w372]
    stop <- w384 stop-if-true
    n207 = Dequeue Element(queue=w386, error in (no error)=w385) -> (queue out=w383:refnum<queue>, element=w382:T6, error out=w384:errorcluster)  [unwired: 1 in, 1 out]
    n208 = Unbundle(w382) -> ("Command"=w381:T7, "Data"=w380:variant)
    n209 = case shown="에러 없음" w384 {
      selector: w384 -> [w398 _]
      tunnel: w383 -> [w397 _]
      tunnel: w381 -> [w396 _]
      tunnel: w380 -> [w395 _]
      tunnel: [w394 _] -> w379
      tunnel: w378 -> [w393 _]
      tunnel: [w392 _] -> w377
      tunnel: w376 -> [w391 _]
      tunnel: [w390 _] -> w375
      tunnel: w374 -> [w389 _]
      tunnel: [w388 _] -> w373
      tunnel: w372 -> [w387 _]
      frame No Error {
        n210 = case shown="\"Scope_Receive\"" w396 {
          tunnel: w398 -> [w408 w433 w508]
          tunnel: w397 -> [_ _ w509]
          tunnel: w395 -> [w409 w434 _]
          tunnel: [w411 w425 _] -> w394
          tunnel: w393 -> [_ w428 _]
          tunnel: [w413 w423 _] -> w392
          tunnel: w391 -> [_ w423 _]
          tunnel: [FALSE w419 _] -> w390
          tunnel: w389 -> [_ w421 _]
          tunnel: [w407 w420 _] -> w388
          tunnel: w387 -> [_ w420 _]
          frame "Scope_Start", Default {
            # "3200Hz"
            # "배열에 삽입 함수를 사용하기 때문에\n빈 배열 상수가 아닌 행을 9개로 초기화"
            # "연결 확인된 센서"
            n211 = Variant To Data(error in=w408, type=bool[] [] ("타입"), Variant=w409) -> (data=w407:bool[])  [unwired: 1 out]
            n212 = local read "Scope_Record Time"() -> (w403:dbl)
            n213 = local read "Auto_Record Time"() -> (w402:dbl)
            n214 = local read "Mode"() -> (w404:enum32{"Auto Playback", "Scope Mode"})
            n215 = Equal?(x=w404, y=enum32{"Auto Playback", "Scope Mode"}."Scope Mode") -> (x = y?=w405:bool)
            n216 = Select(t=w403, s=w405, f=w402) -> (s? t:f=w400:dbl)
            n217 = Initialize Array(0.0 ("원소"), 9 ("차원 크기"), 0 ("차원 크기")) -> (w411:dbl[][])
            "Graph" <- w411
            n218 = Divide(x=w400, y=0.0003125) -> (x/y=w413:dbl)
            "Graph_PP" <- T1 {"S1_Axis"=enum."X Axis", "S1_Value"=0.0, "S2_Axis"=enum."X Axis", "S2_Value"=0.0, "S3_Axis"=enum."X Axis", "S3_Value"=0.0} ("Graph_PP")
          }
          frame "Scope_Receive" {
            (unwired) 0.031 ("y")
            # "Full Resolution일 때 Scale Factor\n센서 스펙 참고"
            n219 = Variant To Data(error in=w433, type=i16[][] [] ("타입"), Variant=w434) -> (data=w431:i16[][])  [unwired: 1 out]
            n220 = Array Size(array=w428) -> (size(s)=w427:i32[])
            n221 = Transpose 2D Array(2D array=w431) -> (transposed array=w430:i16[][])
            n222 = Index Array(array=w427) -> (element #2=w426:i32)  [unwired: 2 in, 1 out]
            n223 = Multiply(x=w430, y=0.0039) -> (x*y=w429:dbl[][])
            n224 = local read "Mode"() -> (w422:enum32{"Auto Playback", "Scope Mode"})
            n225 = Insert Into Array(array=w428, index (col)=w426, new element=w429) -> (w424:dbl[][])  [unwired: 1 in]
            n226 = case shown="\"Scope Mode\"" w422 {
              tunnel: [w436 w444] -> w425
              tunnel: w424 -> [w439 w446]
              tunnel: w423 -> [w438 w445]
              tunnel: "Scope_Trig Type" -> [_ w443]
              tunnel: w421 -> [_ w442]
              tunnel: w420 -> [w435 w441]
              tunnel: [_ w440] -> w419
              frame "Auto Playback", Default {
                n227 = call "(SubVI)Scope_Graph_Array Subset.vi"("length"=w438, "data in"=w439) -> ("data out"=w436:dbl[][])  [unwired: 8 in, 1 out]
                n228 = call "(SubVI)Scope_Peak to Peak.vi"("Activated Ch"=w435, "Data In"=w436) -> ("PP"=w437:T1)  [unwired: 9 in]
                n229 = local write "Graph"(w436) -> ()
                n230 = local write "Graph_PP"(w437) -> ()
              }
              frame "Scope Mode" {
                n231 = case shown="\"Repeat\", \"Single\"" w443 {
                  selector: w443 -> [_ w452]
                  tunnel: w446 -> [w451 w458]
                  tunnel: w445 -> [w450 w453]
                  tunnel: [w448 w457] -> w444
                  tunnel: w442 -> [_ w456]
                  tunnel: w441 -> [w447 w455]
                  tunnel: [_ w454] -> w440
                  frame "None", Default {
                    n232 = call "(SubVI)Scope_Graph_Array Subset.vi"("length"=w450, "data in"=w451) -> ("data out"=w448:dbl[][])  [unwired: 8 in, 1 out]
                    n233 = call "(SubVI)Scope_Peak to Peak.vi"("Activated Ch"=w447, "Data In"=w448) -> ("PP"=w449:T1)  [unwired: 9 in]
                    n234 = local write "Graph"(w448) -> ()
                    n235 = local write "Graph_PP"(w449) -> ()
                  }
                  frame "Repeat", "Single" {
                    n236 = case shown="거짓" w456 {
                      tunnel: w458 -> [w471 w489]
                      tunnel: [w470 w487] -> w457
                      tunnel: w455 -> [w459 w483]
                      tunnel: [w465 w486] -> w454
                      tunnel: w453 -> [w464 w485]
                      tunnel: w452 -> [_ w484]
                      frame False {
                        # "Trigger 확인"
                        # "Trigger 발생 전"
                        n237 = Multiply(x=w464, y="Scope_Pre-trigger") -> (x*y=w466:dbl)
                        n238 = call "(SubVI)Scope_Trigger.vi"("Activated Ch"=w459, "Scope_Trig Level"="Scope_Trig Level", "Scope_Trig Edge"="Scope_Trig Edge", "Scope_Trig Ch"="Scope_Trig Ch", "data in"=w471) -> ("Trigger"=w468:bool, "Trigger Point"=w467:i32, "data out"=w469:dbl[][])  [unwired: 4 in]
                        n239 = case shown="참" w468 {
                          tunnel: w469 -> [w474 w480]
                          tunnel: [w473 w476] -> w470
                          tunnel: w467 -> [_ w482]
                          tunnel: w466 -> [w472 w481]
                          tunnel: [_ TRUE] -> w465
                          tunnel: w459 -> [_ w475]
                          frame False {
                            # "Trigger 발생 전에는\nPre-Trigger 길이 만큼만 유지"
                            n240 = call "(SubVI)Scope_Graph_Array Subset.vi"("length"=w472, "data in"=w474) -> ("data out"=w473:dbl[][])  [unwired: 8 in, 1 out]
                          }
                          frame True {
                            # "Trigger 발생 시점부터\nPre-Trigger 길이까지만 잘라내기"
                            n241 = Subtract(x=w482, y=w481) -> (x-y=w479:dbl)
                            n242 = Array Subset(array=w480, index (col)=w479) -> (w476:dbl[][])  [unwired: 3 in]
                            n243 = call "(SubVI)Scope_Peak to Peak.vi"("Activated Ch"=w475, "Data In"=w476) -> ("PP"=w477:T1)  [unwired: 9 in]
                            n244 = local write "Graph"(w476) -> ()
                            n245 = local write "Graph_PP"(w477) -> ()
                          }
                        }
                      }
                      frame True {
                        # "Trigger 발생 후"
                        n246 = Array Size(array=w489) -> (size(s)=w491:i32[])
                        n247 = Index Array(array=w491) -> (element #2=w490:i32)  [unwired: 2 in, 1 out]
                        n248 = Greater Or Equal?(x=w490, y=w485) -> (x >= y?=w488:bool)
                        n249 = case shown="참" w488 {
                          tunnel: w489 -> [w493 w503]
                          tunnel: w485 -> [_ w502]
                          tunnel: [w493 w500] -> w487
                          tunnel: [TRUE _] -> w486
                          tunnel: w484 -> [_ w499]
                          tunnel: w483 -> [w492 w496]
                          frame False {
                            # "Record Time 길이까지 데이터 모으기"
                            n250 = call "(SubVI)Scope_Peak to Peak.vi"("Activated Ch"=w492, "Data In"=w493) -> ("PP"=w494:T1)  [unwired: 9 in]
                            n251 = local write "Graph"(w493) -> ()
                            n252 = local write "Graph_PP"(w494) -> ()
                          }
                          frame True {
                            # "Trigger\n초기화"
                            # "Record Time 길이까지 잘라내기"
                            n253 = case shown="\"Single\"" w499 {
                              frame "None", Default {
                              }
                              frame "Single" {
                                n254 = property on="Scope_Stop" class="Bool (엄격한)"("Val(Sgnl)"=FALSE ("값(신호)")) -> (error out=w505:errorcluster)  [unwired: 2 in, 1 out]
                                n255 = call "Stall Data Flow.vim"("value in"=w505, "milliseconds to wait"=u32 200) -> ()  [unwired: 2 out]
                              }
                            }
                            n256 = Delete From Array(array=w503, length=w502, index (col)=0 ("비활성화된 인덱스 (열)")) -> (deleted portion=w497:dbl[][], array with subset deleted=w500:dbl[][])  [unwired: 1 in]
                            n257 = call "(SubVI)Scope_Peak to Peak.vi"("Activated Ch"=w496, "Data In"=w497) -> ("PP"=w498:T1)  [unwired: 9 in]
                            n258 = local write "Graph"(w497) -> ()
                            n259 = local write "Graph_PP"(w498) -> ()
                          }
                        }
                      }
                    }
                  }
                }
              }
            }
          }
          frame "Scope_Stop" {
            # "for Auto Playback Mode"
            n260 = Flush Queue(queue=w509, error in (no error)=w508) -> (error out=w507:errorcluster)  [unwired: 2 out]
            n261 = call <vilib>:"Unset Busy.vi"("error in (no error)"=w507) -> ()  [unwired: 10 in, 1 out]
          }
        }
      }
      frame Error {
      }
    }
  }
  n262 = call "Stall Data Flow.vim"("value in"=w67, "milliseconds to wait"=u32 500) -> ("value out"=w38:errorcluster)  [unwired: 1 out]
  n263 = Unregister For Events(event registration refnum=w39) -> ()  [unwired: 1 in, 1 out]
  n264 = Release Queue(queue=w68, error in (no error)=w38) -> ()  [unwired: 1 in, 3 out]
  n265 = Release Queue(queue=w60, error in (no error)=w59) -> ()  [unwired: 1 in, 3 out]
